vi "geve-error_handler.vi"(8 "error in (no error)":errorcluster, 11 "Runtime Data in":T1={"GEVE Ventilator Monitoring Data"={"On/Off"=FALSE, "Error Ack"=FALSE, "bpm"=0.0, "VT"=0.0, "IE"=0.0, "PEEP"=0.0, "Pressure"=0.0, "Plateau Pressure"=0.0, "Motor Position"=0.0, "Alarm P High"=FALSE, "Alarm P Low"=FALSE, "Alarm Init"=FALSE}, "Serial Port Configuration"={"timeout (ms)"=0, "VISA resource name"="", "baud rate"=0, "max expected byte count"=128}, "Serial Read Return Count"=0, "Read Buffer"="", "Communication Timeout?"=FALSE, "com-refs"={"msg-self Q"=refnum, "gui stop event"=refnum}}) -> (0 "error out":errorcluster, 3 "Runtime Data out":T1={"GEVE Ventilator Monitoring Data"={"On/Off"=FALSE, "Error Ack"=FALSE, "bpm"=0.0, "VT"=0.0, "IE"=0.0, "PEEP"=0.0, "Pressure"=0.0, "Plateau Pressure"=0.0, "Motor Position"=0.0, "Alarm P High"=FALSE, "Alarm P Low"=FALSE, "Alarm Init"=FALSE}, "Serial Port Configuration"={"timeout (ms)"=0, "VISA resource name"="", "baud rate"=0, "max expected byte count"=128}, "Serial Read Return Count"=0, "Read Buffer"="", "Communication Timeout?"=FALSE, "com-refs"={"msg-self Q"=refnum, "gui stop event"=refnum}})   [LabVIEW 2018]
doc: "handles errors and treat them depending on error code.\ndefault code :Unknown error.\n Panic. And stop the application (Worker and GUI).\n -1073807339 \nSerial communication timeout error.\nJust clear it and keep listening.\n\n85 :\nScan from the string buffer failed.\nWe've likely received garbage lingering in the buffer.\nDiscard the buffer contents and clear the error.\n\n1:\nScan from the string buffer failed.\nWe've received some weird character.\nDiscard the buffer contents and clear the error.\n\n -1073807343\nConnection to Arduino failed initially.\nEither the Arduino is not connected or the wrong COM port was selected.\nInform the user, then wait a bit, then clear the error to try again.\n\n -1073807194 \nConnection to Arduino lost.\nSomeone must have tripped over the cable.\nInform the user, then wait a bit, then clear the error to try again.\n\n-1073807338\nSomeone must have tripped over the cable.\nInform the user, then wait a bit, then clear the error to try again."
uses:
  geve-runtime_data_cluster.ctl
  geve-monitoring_data_cluster.ctl
  geve-serial_config_cluster.ctl
  geve-com_ref_cluster.ctl
  geve-message_cluster.ctl
  <vilib>/Utility/error.llb/DialogType.ctl
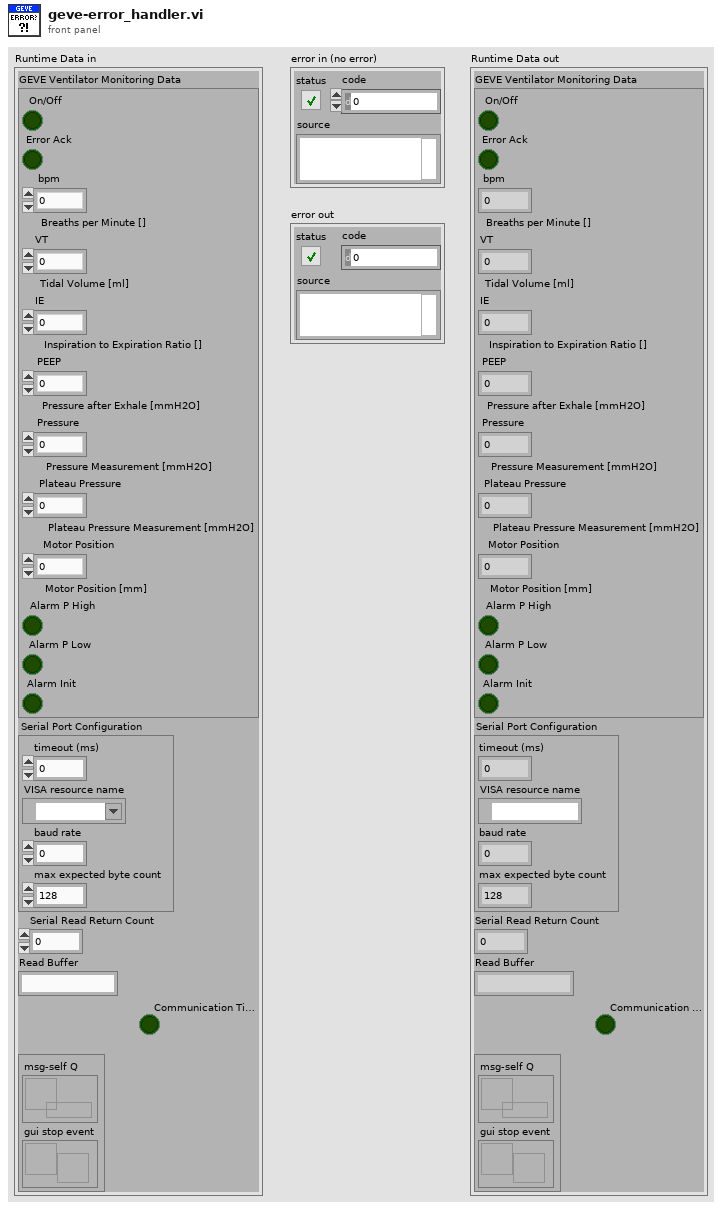
[diagram p1: front panel]
types:
  T1 = typedef "geve-runtime_data_cluster.ctl" = cluster{"GEVE Ventilator Monitoring Data":T2, "Serial Port Configuration":T3, "Serial Read Return Count":u32, "Read Buffer":string, "Communication Timeout?":bool, "com-refs":T4}
  T2 = typedef "geve-monitoring_data_cluster.ctl" = cluster{"On/Off":bool, "Error Ack":bool, "bpm":dbl, "VT":dbl, "IE":dbl, "PEEP":dbl, "Pressure":dbl, "Plateau Pressure":dbl, "Motor Position":dbl, "Alarm P High":bool, "Alarm P Low":bool, "Alarm Init":bool}
  T3 = typedef "geve-serial_config_cluster.ctl" = cluster{"timeout (ms)":u32, "VISA resource name":refnum<visa-resource-name>, "baud rate":u32, "max expected byte count":u32}
  T4 = typedef "geve-com_ref_cluster.ctl" = cluster{"msg-self Q":refnum<queue>, "gui stop event":refnum<user-event>}
  T5 = typedef "DialogType.ctl" = u16
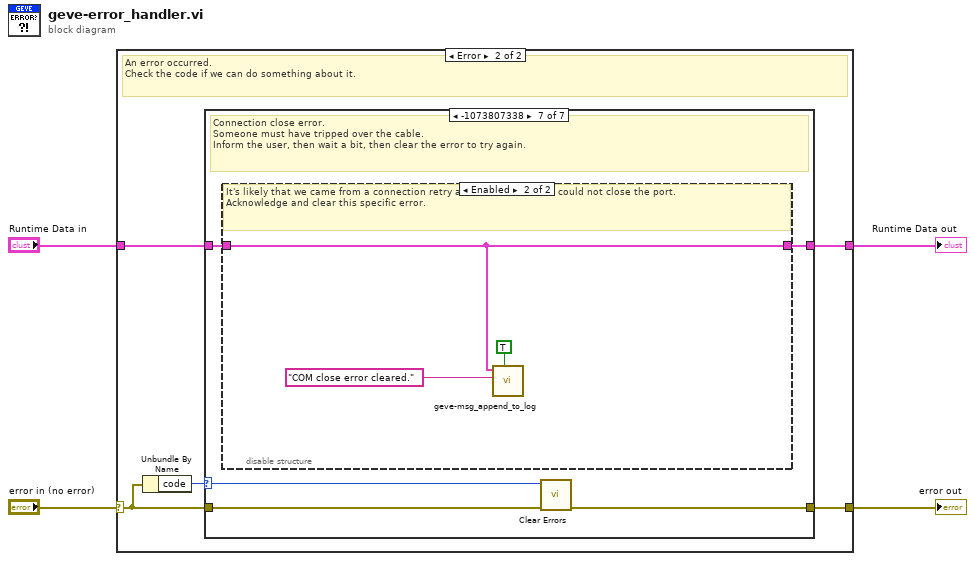
[diagram p0: block diagram]
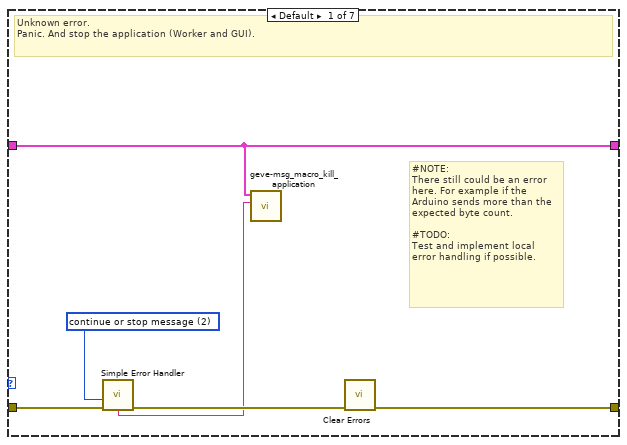
[diagram p3: hidden frame]
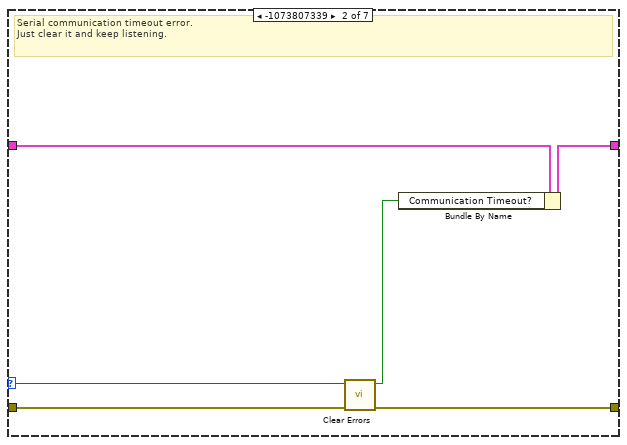
[diagram p4: hidden frame]
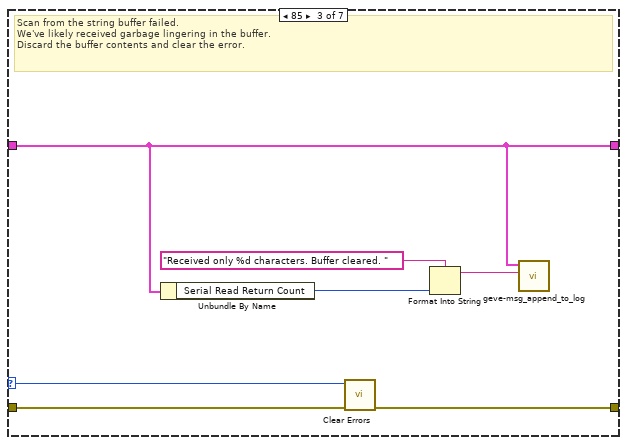
[diagram p5: hidden frame]
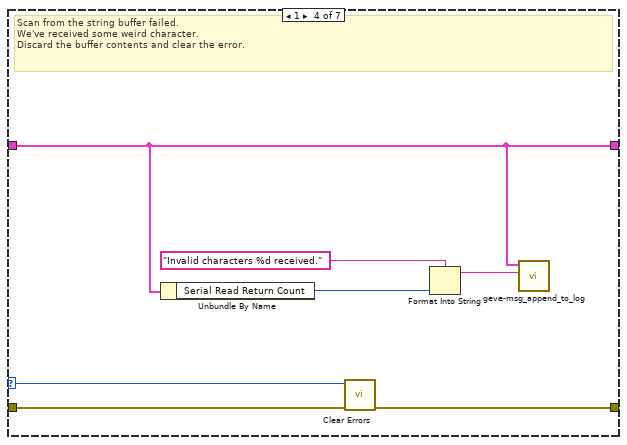
[diagram p6: hidden frame]
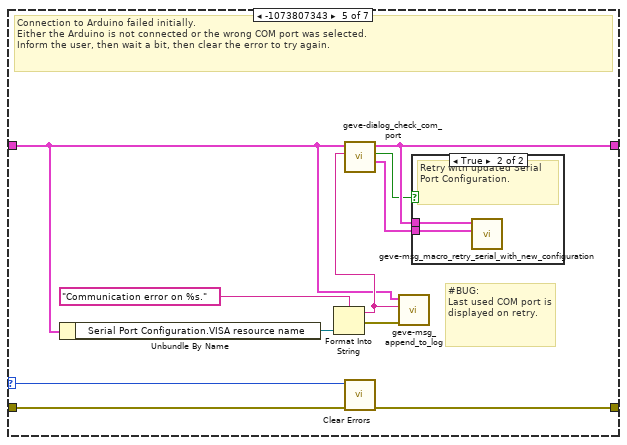
[diagram p7: hidden frame]
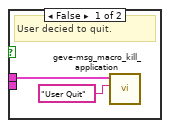
[diagram p8: hidden frame]
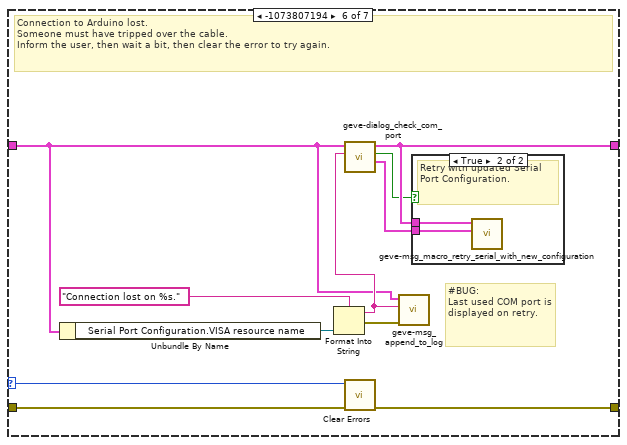
[diagram p9: hidden frame]
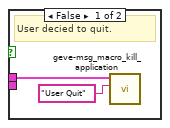
[diagram p10: hidden frame]
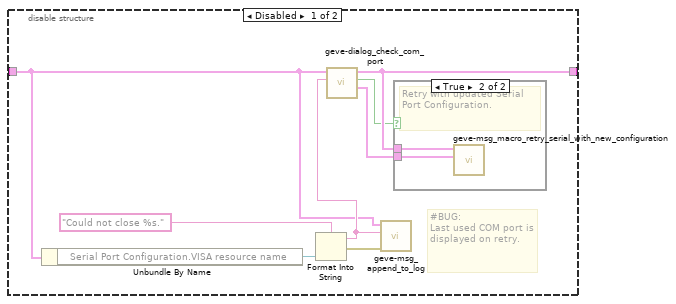
[diagram p11: hidden frame]
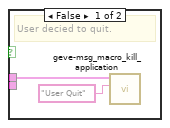
[diagram p12: hidden frame]
diagram:
  n1 = case shown="Error" "error in (no error)" {
    selector: "error in (no error)" -> [w6 w10]
    tunnel: [w6 w11] -> w4
    tunnel: [w5 w8] -> w2
    tunnel: "Runtime Data in" -> [w5 w7]
    frame No Error {
      # "All is good."
    }
    frame Error {
      # "An error occurred.\nCheck the code if we can do something about it."
      n2 = Unbundle By Name(w10) -> ("code"=w9:i32)
      n3 = case shown="-1073807338" w9 {
        selector: w9 -> [_ w19 w25 w33 w38 w53 w68]
        tunnel: w10 -> [w15 w23 w24 w32 w46 w62 w71]
        tunnel: [w17 w22 w30 w37 w48 w63 w72] -> w11
        tunnel: [w12 w20 w29 w36 w44 w60 w70] -> w8
        tunnel: w7 -> [w12 w21 w29 w36 w39 w55 w69]
        frame Default {
          w16 = T5 2 items=["no dialog", "OK message", "continue or stop message", "OK message + warnings", "continue/stop + warnings"] ("type of dialog (OK msg:1)")
          # "#NOTE:\nThere still could be an error here. For example if the Arduino sends more than the expected byte count.\n\n#TODO:\nTest and implement local error handling if possible."
          # "Unknown error.\nPanic. And stop the application (Worker and GUI)."
          n4 = call <vilib>:"Simple Error Handler.vi"("type of dialog (OK msg:1)"=w16, "error in (no error)"=w15) -> ("error out"=w14:errorcluster, "message"=w13:string)  [unwired: 3 in, 3 out]
          n5 = call "geve-msg_macro_kill_application.vi"("Kill log message"=w13, "Runtime Data in"=w12) -> ()  [unwired: 10 in]
          n6 = call <vilib>:"Clear Errors.vi"("error in (no error)"=w14) -> ("error out"=w17:errorcluster)  [unwired: 5 in, 1 out]
        }
        frame -1073807339 {
          # "Serial communication timeout error.\nJust clear it and keep listening."
          n7 = call <vilib>:"Clear Errors.vi"("error in (no error)"=w23, "specific error code to clear (0: all)"=w19) -> ("error out"=w22:errorcluster, "specific error cleared?"=w18:bool)  [unwired: 4 in]
          n8 = Bundle By Name(cluster=w21, "Communication Timeout?"=w18) -> (w20:T1)
        }
        frame 85 {
          # "Scan from the string buffer failed.\nWe've likely received garbage lingering in the buffer.\nDiscard the buffer contents and clear the error."
          n9 = Unbundle By Name(w29) -> ("Serial Read Return Count"=w27:u32)
          n10 = call <vilib>:"Clear Errors.vi"("error in (no error)"=w24, "specific error code to clear (0: all)"=w25) -> ("error out"=w30:errorcluster)  [unwired: 4 in, 1 out]
          n11 = Format Into String(format string="Received only %d characters. Buffer cleared. " ("string"), w27) -> (resulting string=w26:string)  [unwired: 2 in, 1 out]
          n12 = call "geve-msg_append_to_log.vi"("Status Message"=w26, "Runtime Data"=w29) -> ()  [unwired: 8 in, 2 out]
        }
        frame 1 {
          # "Scan from the string buffer failed.\nWe've received some weird character.\nDiscard the buffer contents and clear the error."
          n13 = Unbundle By Name(w36) -> ("Serial Read Return Count"=w35:u32)
          n14 = call <vilib>:"Clear Errors.vi"("error in (no error)"=w32, "specific error code to clear (0: all)"=w33) -> ("error out"=w37:errorcluster)  [unwired: 4 in, 1 out]
          n15 = Format Into String(format string="Invalid characters %d received." ("string"), w35) -> (resulting string=w34:string)  [unwired: 2 in, 1 out]
          n16 = call "geve-msg_append_to_log.vi"("Status Message"=w34, "Runtime Data"=w36) -> ()  [unwired: 8 in, 2 out]
        }
        frame -1073807343 {
          # "#BUG:\nLast used COM port is displayed on retry."
          # "Connection to Arduino failed initially.\nEither the Arduino is not connected or the wrong COM port was selected.\nInform the user, then wait a bit, then clear the error to try again."
          n17 = Unbundle By Name(w39) -> ("Serial Port Configuration.VISA resource name"=w47:refnum<visa-resource-name>)
          n18 = Format Into String(format string="Communication error on %s." ("string"), w47) -> (resulting string=w41:string, error out=w40:errorcluster)  [unwired: 2 in]
          n19 = call "geve-dialog_check_com_port.vi"("Application Message"=w41, "Runtime Data in"=w39) -> ("Updated Serial Port Configuration"=w42:T3, "Retry?"=w43:bool, "Runtime Data out"=w44:T1)  [unwired: 7 in]
          n20 = call <vilib>:"Clear Errors.vi"("error in (no error)"=w46, "specific error code to clear (0: all)"=w38) -> ("error out"=w48:errorcluster)  [unwired: 4 in, 1 out]
          n21 = call "geve-msg_append_to_log.vi"("error in (no error)"=w40, "Status Message"=w41, "Runtime Data"=w39) -> ()  [unwired: 7 in, 2 out]
          n22 = case shown="True" w43 {
            tunnel: w44 -> [w49 w52]
            tunnel: w42 -> [_ w51]
            frame False {
              # "User decied to quit."
              n23 = call "geve-msg_macro_kill_application.vi"("Kill log message"="User Quit", "Runtime Data in"=w49) -> ()  [unwired: 10 in]
            }
            frame True {
              # "Retry with updated Serial Port Configuration."
              n24 = call "geve-msg_macro_retry_serial_with_new_configuration.vi"("Serial Port Configuration"=w51, "Runtime Data in"=w52) -> ()  [unwired: 10 in]
            }
          }
        }
        frame -1073807194 {
          # "#BUG:\nLast used COM port is displayed on retry."
          # "Connection to Arduino lost.\nSomeone must have tripped over the cable.\nInform the user, then wait a bit, then clear the error to try again."
          n25 = Unbundle By Name(w55) -> ("Serial Port Configuration.VISA resource name"=w54:refnum<visa-resource-name>)
          n26 = Format Into String(format string="Connection lost on %s." ("string"), w54) -> (resulting string=w57:string, error out=w56:errorcluster)  [unwired: 2 in]
          n27 = call "geve-dialog_check_com_port.vi"("Application Message"=w57, "Runtime Data in"=w55) -> ("Updated Serial Port Configuration"=w58:T3, "Retry?"=w59:bool, "Runtime Data out"=w60:T1)  [unwired: 7 in]
          n28 = call <vilib>:"Clear Errors.vi"("error in (no error)"=w62, "specific error code to clear (0: all)"=w53) -> ("error out"=w63:errorcluster)  [unwired: 4 in, 1 out]
          n29 = call "geve-msg_append_to_log.vi"("error in (no error)"=w56, "Status Message"=w57, "Runtime Data"=w55) -> ()  [unwired: 7 in, 2 out]
          n30 = case shown="True" w59 {
            tunnel: w60 -> [w64 w67]
            tunnel: w58 -> [_ w66]
            frame False {
              # "User decied to quit."
              n31 = call "geve-msg_macro_kill_application.vi"("Kill log message"="User Quit", "Runtime Data in"=w64) -> ()  [unwired: 10 in]
            }
            frame True {
              # "Retry with updated Serial Port Configuration."
              n32 = call "geve-msg_macro_retry_serial_with_new_configuration.vi"("Serial Port Configuration"=w66, "Runtime Data in"=w67) -> ()  [unwired: 10 in]
            }
          }
        }
        frame -1073807338 {
          # "Connection close error.\nSomeone must have tripped over the cable.\nInform the user, then wait a bit, then clear the error to try again."
          n33 = disable-structure shown="Enabled" {
            disable-tunnel: [w79 w87] -> w70
            disable-tunnel: w69 -> [w74 w87]
            frame Disabled {
              # "#BUG:\nLast used COM port is displayed on retry."
              n34 = Unbundle By Name(w74) -> ("Serial Port Configuration.VISA resource name"=w73:refnum<visa-resource-name>)
              n35 = Format Into String(format string="Could not close %s." ("string"), w73) -> (resulting string=w76:string, error out=w75:errorcluster)  [unwired: 2 in]
              n36 = call "geve-dialog_check_com_port.vi"("Application Message"=w76, "Runtime Data in"=w74) -> ("Updated Serial Port Configuration"=w77:T3, "Retry?"=w78:bool, "Runtime Data out"=w79:T1)  [unwired: 7 in]
              n37 = call "geve-msg_append_to_log.vi"("error in (no error)"=w75, "Status Message"=w76, "Runtime Data"=w74) -> ()  [unwired: 7 in, 2 out]
              n38 = case shown="True" w78 {
                tunnel: w79 -> [w81 w84]
                tunnel: w77 -> [_ w83]
                frame False {
                  # "User decied to quit."
                  n39 = call "geve-msg_macro_kill_application.vi"("Kill log message"="User Quit", "Runtime Data in"=w81) -> ()  [unwired: 10 in]
                }
                frame True {
                  # "Retry with updated Serial Port Configuration."
                  n40 = call "geve-msg_macro_retry_serial_with_new_configuration.vi"("Serial Port Configuration"=w83, "Runtime Data in"=w84) -> ()  [unwired: 10 in]
                }
              }
            }
            frame Enabled {
              # "It's likely that we came from a connection retry and we know that we could not close the port.\nAcknowledge and clear this specific error."
              n41 = call "geve-msg_append_to_log.vi"("Priority"=TRUE, "Status Message"="COM close error cleared.", "Runtime Data"=w87) -> ()  [unwired: 7 in, 2 out]
            }
          }
          n42 = call <vilib>:"Clear Errors.vi"("error in (no error)"=w71, "specific error code to clear (0: all)"=w68) -> ("error out"=w72:errorcluster)  [unwired: 4 in, 1 out]
        }
      }
    }
  }
  "error out" <- w4
  "Runtime Data out" <- w2
